vi "anda_dist_x.vi"() -> ()   [LabVIEW 2016]
uses:
  <vilib>/NXT/Subs/LVHSConnector.ctl
  <vilib>/NXT/LegoClasses/BrickReference/BrickReference.lvclass
  <vilib>/NXT/Block Support/NXT_OutputPort.ctl
  <vilib>/NXT/Dual Mode Library/Motors/ResetMotor.vi
  <vilib>/NXT/Dual Mode Library/Motors/Rotation.vi
  <vilib>/NXT/NXTIO Xnodes/AddressXNode/NXTIOAddress.xnode
panel:
  in  "KE":dbl=-0.0356
  in  "dist (cm)":dbl
  in  "NXT/EV3":T1
  out "NXT/EV3 2":T1
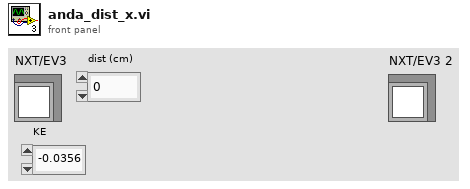
[diagram p1: front panel]
types:
  T1 = typedef "LVHSConnector.ctl" = refnum<class "BrickReference.lvclass">
  T2 = typedef "NXT_OutputPort.ctl" = u8
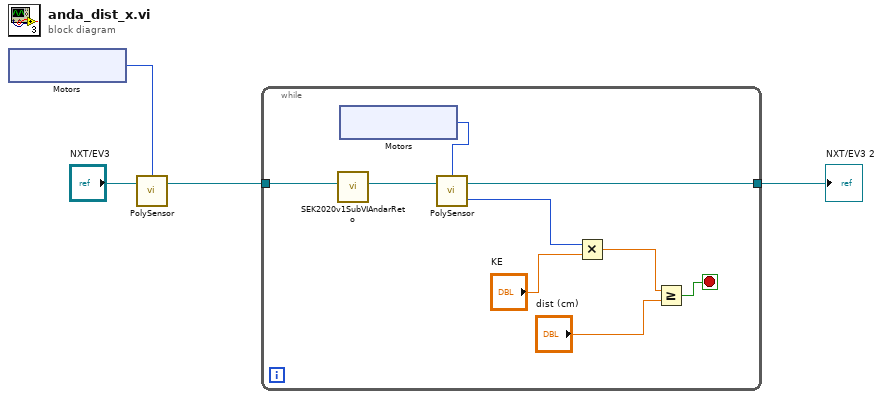
[diagram p0: block diagram]
diagram:
  n1 = xnode "Motors"() -> ("Motor"=w3:T2)
  n2 = call-poly <vilib>:"PolySensor.vi"("NXT/EV3"="NXT/EV3", "Port (All Ports)"=w3) -> ("NXT/EV3"=w2:T1)  [unwired: 2 out]
  n3 = while {
    tunnel: w2 -> [w10]
    tunnel: [w13] -> w1
    stop <- w11 stop-if-true
    n4 = call "SEK2020v1SubVIAndarReto.vi"("NXT/EV3"=w10) -> ("NXT/EV3 2"=w9:T1)  [unwired: 9 in]
    n5 = xnode "Motors"() -> ("Motor"=w8:T2)
    n6 = call-poly <vilib>:"PolySensor.vi"("NXT/EV3"=w9, "Port (Port A)"=w8) -> ("Angle of Rotation"=w7:i32, "NXT/EV3"=w13:T1)  [unwired: 1 out]
    n7 = Multiply(x=w7, y="KE") -> (x*y=w6:dbl)
    n8 = Greater Or Equal?(x=w6, y="dist (cm)") -> (x >= y?=w11:bool)
  }
  "NXT/EV3 2" <- w1
